vi "countspersec_LT.vi"(1 "1D PH data":u32[](array[numeric])) -> (0 "Avg cts/s":dbl)   [LabVIEW 2015]
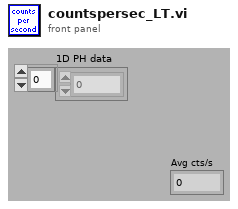
[diagram p1: front panel]
types:
  T1 = cluster{"initialized":bool, "devidx":i32, "Ch0 Level":i32, "Ch0 ZeroX":i32, "Ch1 Level":i32, "Ch1 ZeroX":i32, "sync rate":i32, "resolution":i32, "acq time":i32, "acq rate":i32, "# bins":u32, "Bin size":enum16{"1", "2", "4", "8", "16", "32", "64", "128"}, "min photons":u32, "truncate":u32}
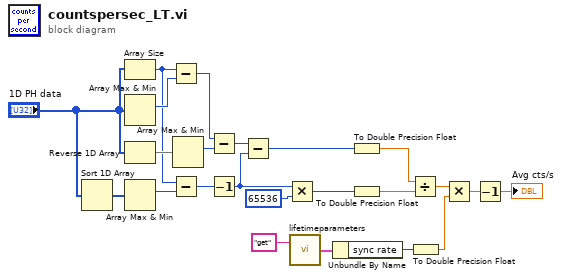
[diagram p0: block diagram]
diagram:
  n1 = Sort 1D Array(array="1D PH data") -> (sorted array=w14:u32[])
  n2 = Array Size(array="1D PH data") -> (size(s)=w11:i32)
  n3 = Array Max & Min(array="1D PH data") -> (max index (indices)=w15:i32)  [unwired: 3 out]
  n4 = Reverse 1D Array(array="1D PH data") -> (reversed array=w18:u32[])
  n5 = Array Max & Min(array=w14) -> (max index (indices)=w13:i32)  [unwired: 3 out]
  n6 = Subtract(x=w11, y=w15) -> (x-y=w17:i32)
  n7 = Subtract(x=w11, y=w13) -> (x-y=w12:i32)
  n8 = Array Max & Min(array=w18) -> (max index (indices)=w16:i32)  [unwired: 3 out]
  n9 = Subtract(x=w17, y=w16) -> (x-y=w10:i32)
  n10 = Decrement(x=w12) -> (x-1=w3:i32)
  n11 = Subtract(x=w10, y=w3) -> (x-y=w6:i32)
  n12 = Multiply(x=w3, y=65536 ("x")) -> (x*y=w5:i32)
  n13 = call "lifetimeparameters.vi"("command"="get") -> ("Params out"=w20:T1)  [unwired: 1 in]
  n14 = Unbundle By Name(w20) -> ("sync rate"=w19:i32)
  n15 = To Double Precision Float(number=w6) -> (double precision float=w9:dbl)
  n16 = To Double Precision Float(number=w5) -> (double precision float=w8:dbl)
  n17 = Divide(x=w9, y=w8) -> (x/y=w7:dbl)
  n18 = To Double Precision Float(number=w19) -> (double precision float=w23:dbl)
  n19 = Multiply(x=w7, y=w23) -> (x*y=w22:dbl)
  n20 = Decrement(x=w22) -> (x-1=→"Avg cts/s":dbl)
